vi "ReadBundler.vi"(1 "reference":refnum<vi>) -> (0 "Bundler":T5)   [LabVIEW 2013]
uses:
  <vilib>/Utility/miscctls.llb/LVBoundsTypeDef.ctl
  <vilib>/Utility/miscctls.llb/LVPositionTypeDef.ctl
  <vilib>/Utility/miscctls.llb/LVRectTypeDef.ctl
  <vilib>/Utility/miscctls.llb/LVBreakpointStatusEnum.ctl
panel:
  out "error out 22":errorcluster
  out "error out 21":errorcluster
  out "error out 20":errorcluster
  out "error out 19":errorcluster
  out "error out 18":errorcluster
  out "error out 17":errorcluster
  out "error out 16":errorcluster
  out "error out 15":errorcluster
  out "error out 14":errorcluster
  out "error out 13":errorcluster
  out "error out 12":errorcluster
  out "error out 11":errorcluster
  out "error out 10":errorcluster
  out "error out 9":errorcluster
  out "error out 8":errorcluster
  out "error out 7":errorcluster
  out "error out 6":errorcluster
  out "error out 5":errorcluster
  out "error out 4":errorcluster
  out "error out 3":errorcluster
  out "error out 2":errorcluster
  out "error out":errorcluster
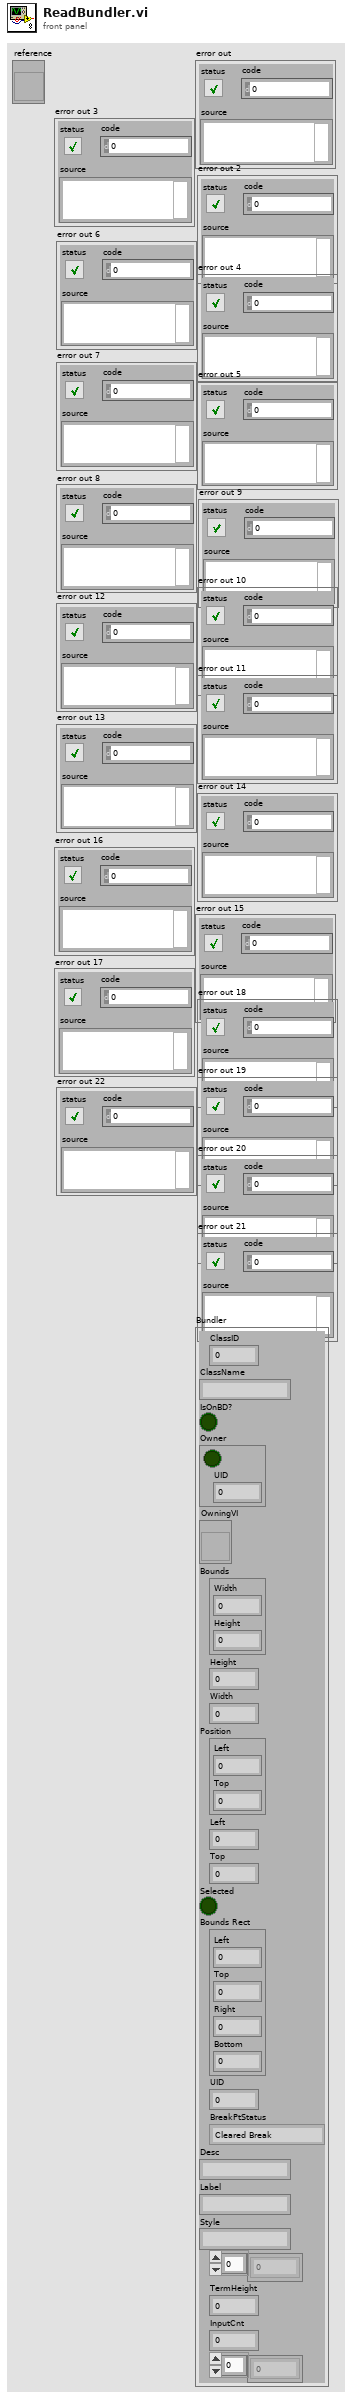
[diagram p1: front panel]
types:
  T1 = typedef "LVBoundsTypeDef.ctl" = cluster{"Width":u32, "Height":u32}
  T2 = typedef "LVPositionTypeDef.ctl" = cluster{"Left":i32, "Top":i32}
  T3 = typedef "LVRectTypeDef.ctl" = cluster{"Left":i16, "Top":i16, "Right":i16, "Bottom":i16}
  T4 = typedef "LVBreakpointStatusEnum.ctl" = enum8{"Cleared Break", "Enabled Break", "Disabled Break"}
  T5 = cluster{"ClassID":u32, "ClassName":string, "IsOnBD?":bool, "Owner":cluster{bool, "UID":i32}, "OwningVI":refnum<vi>, "Bounds":T1, "Height":u32, "Width":u32, "Position":T2, "Left":i32, "Top":i32, "Selected":bool, "Bounds Rect":T3, "UID":i32, "BreakPtStatus":T4, "Desc":string, "Label":string, "Style":string, "Terms[]":i32[], "TermHeight":i32, "InputCnt":i32, "InputTerms[]":i32[]}
  T6 = cluster{"ClassID":u32, "ClassName":string, "IsOnBD?":bool, "Cluster":cluster{bool, "UID":i32}, "OwningVI":refnum<vi>, "Bounds":T1, "Height":u32, "Width":u32, "Position":T2, "Left":i32, "Top":i32, "Selected":bool, "Bounds Rect":T3, "UID":i32, "BreakPtStatus":T4, "Desc":string, "Text":string, "Style":string, i32[], "TermHeight":i32, "InputCnt":i32, i32[]}
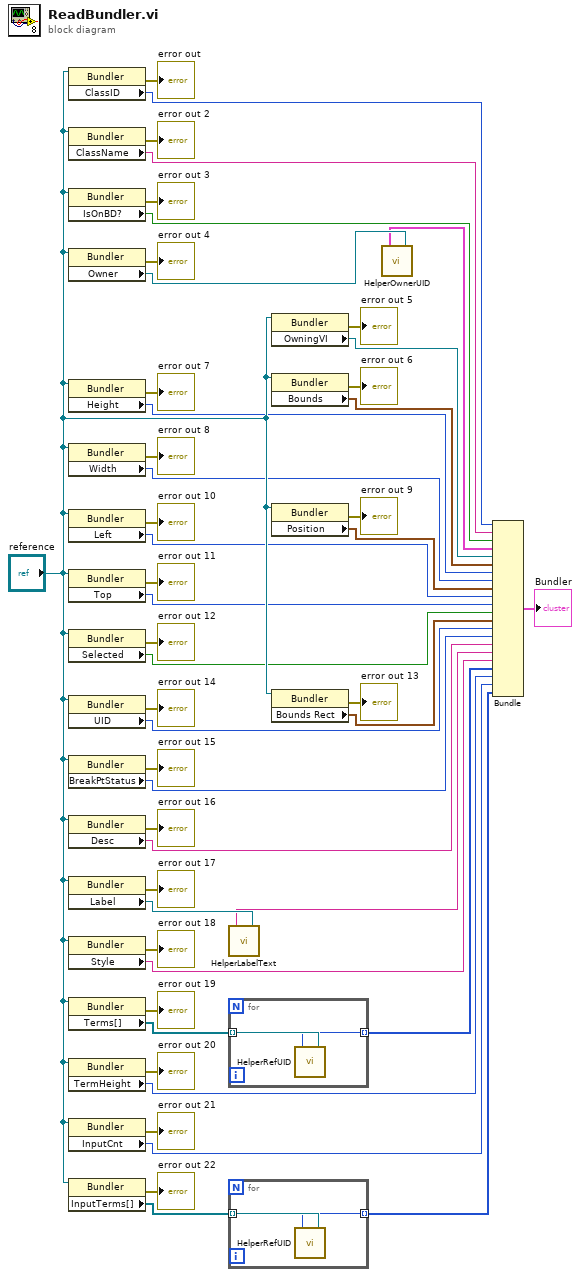
[diagram p0: block diagram]
diagram:
  n1 = property class="Bundler"(reference="reference") -> (error out=→"error out":errorcluster, "ClassID"=w48:u32)  [unwired: 1 in, 1 out]
  n2 = property class="Bundler"(reference="reference") -> (error out=→"error out 2":errorcluster, "ClassName"=w46:string)  [unwired: 1 in, 1 out]
  n3 = property class="Bundler"(reference="reference") -> (error out=→"error out 3":errorcluster, "IsOnBD?"=w44:bool)  [unwired: 1 in, 1 out]
  n4 = property class="Bundler"(reference="reference") -> (error out=→"error out 4":errorcluster, "Owner"=w42:refnum<vi>)  [unwired: 1 in, 1 out]
  n5 = property class="Bundler"(reference="reference") -> (error out=→"error out 7":errorcluster, "Height"=w35:u32)  [unwired: 1 in, 1 out]
  n6 = property class="Bundler"(reference="reference") -> (error out=→"error out 8":errorcluster, "Width"=w33:u32)  [unwired: 1 in, 1 out]
  n7 = property class="Bundler"(reference="reference") -> (error out=→"error out 10":errorcluster, "Left"=w29:i32)  [unwired: 1 in, 1 out]
  n8 = property class="Bundler"(reference="reference") -> (error out=→"error out 11":errorcluster, "Top"=w27:i32)  [unwired: 1 in, 1 out]
  n9 = property class="Bundler"(reference="reference") -> (error out=→"error out 12":errorcluster, "Selected"=w25:bool)  [unwired: 1 in, 1 out]
  n10 = property class="Bundler"(reference="reference") -> (error out=→"error out 14":errorcluster, "UID"=w21:i32)  [unwired: 1 in, 1 out]
  n11 = property class="Bundler"(reference="reference") -> (error out=→"error out 15":errorcluster, "BreakPtStatus"=w19:T4)  [unwired: 1 in, 1 out]
  n12 = property class="Bundler"(reference="reference") -> (error out=→"error out 16":errorcluster, "Desc"=w17:string)  [unwired: 1 in, 1 out]
  n13 = property class="Bundler"(reference="reference") -> (error out=→"error out 17":errorcluster, "Label"=w15:refnum<vi>)  [unwired: 1 in, 1 out]
  n14 = property class="Bundler"(reference="reference") -> (error out=→"error out 18":errorcluster, "Style"=w12:string)  [unwired: 1 in, 1 out]
  n15 = property class="Bundler"(reference="reference") -> (error out=→"error out 19":errorcluster, "Terms[]"=w10:refnum<vi>[])  [unwired: 1 in, 1 out]
  n16 = property class="Bundler"(reference="reference") -> (error out=→"error out 20":errorcluster, "TermHeight"=w7:i32)  [unwired: 1 in, 1 out]
  n17 = property class="Bundler"(reference="reference") -> (error out=→"error out 21":errorcluster, "InputCnt"=w5:i32)  [unwired: 1 in, 1 out]
  n18 = property class="Bundler"(reference="reference") -> (error out=→"error out 22":errorcluster, "InputTerms[]"=w3:refnum<vi>[])  [unwired: 1 in, 1 out]
  n19 = call "HelperLabelText.vi"("Text in"=w15) -> ("Text"=w14:string)
  n20 = for {
    tunnel: w10 -> [w52] mode=indexing
    tunnel: [w51] -> w9 mode=indexing
    n21 = call "HelperRefUID.vi"("Text in"=w52) -> ("UID"=w51:i32)
  }
  n22 = for {
    tunnel: w3 -> [w54] mode=indexing
    tunnel: [w53] -> w2 mode=indexing
    n23 = call "HelperRefUID.vi"("Text in"=w54) -> ("UID"=w53:i32)
  }
  n24 = property class="Bundler"(reference="reference") -> (error out=→"error out 5":errorcluster, "OwningVI"=w39:refnum<vi>)  [unwired: 1 in, 1 out]
  n25 = property class="Bundler"(reference="reference") -> (error out=→"error out 6":errorcluster, "Bounds"=w37:T1)  [unwired: 1 in, 1 out]
  n26 = property class="Bundler"(reference="reference") -> (error out=→"error out 9":errorcluster, "Position"=w31:T2)  [unwired: 1 in, 1 out]
  n27 = property class="Bundler"(reference="reference") -> (error out=→"error out 13":errorcluster, "Bounds Rect"=w23:T3)  [unwired: 1 in, 1 out]
  n28 = call "HelperOwnerUID.vi"("Generic in"=w42) -> ("Cluster"=w41:cluster{bool, "UID":i32})
  n29 = Bundle("ClassID"=w48, "ClassName"=w46, "IsOnBD?"=w44, "Cluster"=w41, "OwningVI"=w39, "Bounds"=w37, "Height"=w35, "Width"=w33, "Position"=w31, "Left"=w29, "Top"=w27, "Selected"=w25, "Bounds Rect"=w23, "UID"=w21, "BreakPtStatus"=w19, "Desc"=w17, "Text"=w14, "Style"=w12, w9, "TermHeight"=w7, "InputCnt"=w5, w2) -> (→"Bundler":T6)  [unwired: 1 in]
